vi "Erase Background.vi"(9 "draw options":T1={"Text Color"=16777238, "Wing Color"=16751616, "Dial Outline Color"=13816530, "Sky Color"=3381759, "Ground Color"=8213043, "Horizon Line Color"=16777225, "Outline Color"=0, "Dial Background Color"=5987163, "Draw Wings"=TRUE, "Draw Text"=TRUE, "Font Name"="Helvetica", "Angle units"=enum."Degrees"}, 10 "draw area state in":T3, 11 "picture in":picture) -> (3 "picture out":picture)   [LabVIEW 2017, in "NI_Robotics_Attitude Picture.lvlib"]
uses:
  <vilib>/robotics/Controls/Attitude Indicator/Attitude Picture/NI_Robotics_Attitude Picture.lvlib
  <vilib>/robotics/Controls/Attitude Indicator/Attitude Picture/Draw Area State.ctl
  <vilib>/Utility/miscctls.llb/LVBoundsTypeDef.ctl
  <vilib>/robotics/Controls/Attitude Indicator/Attitude Picture/Draw Options.ctl
  <vilib>/robotics/Controls/Utilities/Angle Units.ctl
  <vilib>/robotics/Controls/Utilities/NI_Robotics_Control Utilities.lvlib
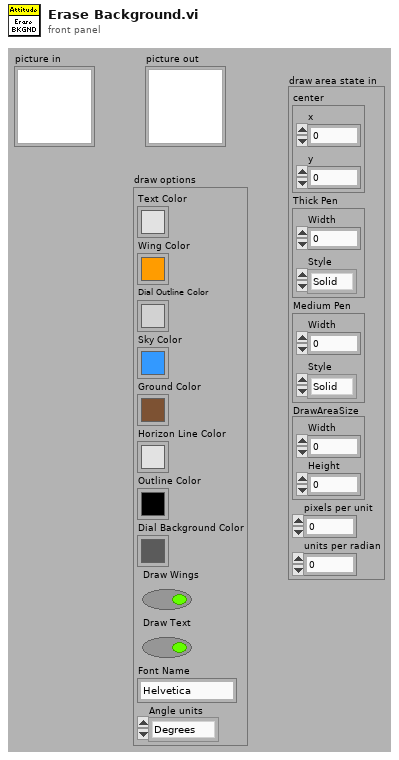
[diagram p1: front panel]
types:
  T1 = typedef "NI_Robotics_Attitude Picture.lvlib/Draw Options.ctl" = cluster{"Text Color":u32, "Wing Color":u32, "Dial Outline Color":u32, "Sky Color":u32, "Ground Color":u32, "Horizon Line Color":u32, "Outline Color":u32, "Dial Background Color":u32, "Draw Wings":bool, "Draw Text":bool, "Font Name":string, "Angle units":T2}
  T2 = typedef "NI_Robotics_Control Utilities.lvlib/Angle Units.ctl" = enum16{"Radians", "Degrees"}
  T3 = typedef "NI_Robotics_Attitude Picture.lvlib/Draw Area State.ctl" = cluster{"center":cluster{"x":i16, "y":i16}, "Thick Pen":cluster{"Width":u16, "Style":enum32{"Solid", "Dash", "Dot", "DashDot", "DashDotDot"}}, "Medium Pen":cluster{"Width":u16, "Style":enum32{"Solid", "Dash", "Dot", "DashDot", "DashDotDot"}}, "DrawAreaSize":T4, "pixels per unit":dbl, "units per radian":dbl}
  T4 = typedef "LVBoundsTypeDef.ctl" = cluster{"Width":u32, "Height":u32}
  T5 = cluster{"left":i16, "top":i16, "right":i16, "bottom":i16}
  T6 = cluster{"Width":u16, "Style":enum32{"Solid", "Dash", "Dot", "DashDot", "DashDotDot"}}
  T7 = typedef "imagedata.ctl" = cluster{"image type":i32, "image depth":i32, "image":u8[], "mask":u8[], "colors":u32[], "Rectangle":cluster{"left":i16, "top":i16, "right":i16, "bottom":i16}}
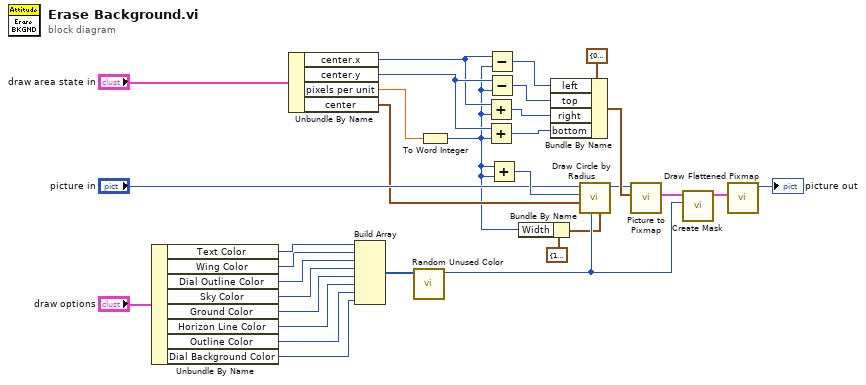
[diagram p0: block diagram]
diagram:
  n1 = Unbundle By Name("draw options") -> ("Text Color"=w13:u32, "Wing Color"=w12:u32, "Dial Outline Color"=w11:u32, "Sky Color"=w10:u32, "Ground Color"=w9:u32, "Horizon Line Color"=w8:u32, "Outline Color"=w7:u32, "Dial Background Color"=w6:u32)
  n2 = Unbundle By Name("draw area state in") -> ("center.x"=w25:i16, "center.y"=w26:i16, "pixels per unit"=w3:dbl, "center"=w2:cluster{"x":i16, "y":i16})
  n3 = Build Array(w13, w12, w11, w10, w9, w8, w7, w6) -> (w5:u32[])
  n4 = call <vilib>:"Random Unused Color.vi"("existing colors"=w5) -> ("new color"=w17:u32)  [unwired: 10 in]
  n5 = To Word Integer(number=w3) -> (16bit integer=w1:i16)
  n6 = Add(x=w25, y=w1) -> (x+y=w29:i16)
  n7 = Add(x=w26, y=w1) -> (x+y=w30:i16)
  n8 = Subtract(x=w25, y=w1) -> (x-y=w27:i16)
  n9 = Subtract(x=w26, y=w1) -> (x-y=w28:i16)
  n10 = Add(x=w1, y=w1) -> (x+y=w19:i16)
  n11 = Bundle By Name(cluster=T6 {"Width"=1000, "Style"=enum."Solid"} ("pen"), "Width"=w1) -> (w15:T6)
  n12 = Bundle By Name(cluster=T5 {"left"=0, "top"=0, "right"=0, "bottom"=0} ("rect"), "left"=w27, "top"=w28, "right"=w29, "bottom"=w30) -> (w31:T5)
  n13 = call <vilib>:"Draw Circle by Radius.vi"("pen"=w15, "color(black)"=w17, "pixel center"=w2, "radius"=w19, "picture"="picture in") -> ("new picture"=w20:picture)  [unwired: 6 in]
  n14 = call <vilib>:"Picture to Pixmap.vi"("rect"=w31, "picture"=w20) -> ("image data"=w21:T7)  [unwired: 8 in, 1 out]
  n15 = call <vilib>:"Create Mask.vi"("Mask Color (Black)"=w17, "image data"=w21) -> ("image data"=w22:T7)  [unwired: 9 in]
  n16 = call <vilib>:"Draw Flattened Pixmap.vi"("image data"=w22) -> ("new picture"=→"picture out":picture)  [unwired: 8 in]
